vi "data-plotter.vi"() -> ()   [LabVIEW 2020]
uses:
  <vilib>/Utility/file.llb/Read Delimited Spreadsheet (DBL).vi
  <vilib>/Utility/file.llb/Read Delimited Spreadsheet (string).vi
panel:
  in  "文字列":string
  out "header row":string[](array[string]) caption="Header (1st row)"
  out "Graph":cluster{dbl[], dbl[]}(graph)
  in  "Y axis":i32
  in  "X axis":i32
  out "error out":errorcluster caption="エラー出力"
  in  "delimiter (\\t)":string="\t" caption="デリミタ (\\t)"
  in  "format (%.3f)":string="%.3f" caption="形式文字列 (%.3f)"
  in  "How many header rows?":i32
  in  "file path (dialog if empty)":path caption="ファイルパス (空の場合はダイアログ)"
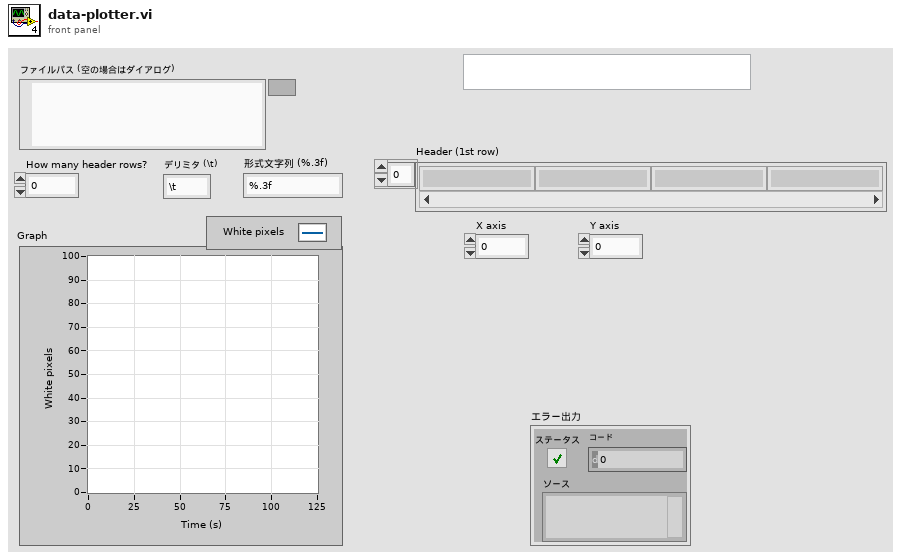
[diagram p1: front panel]
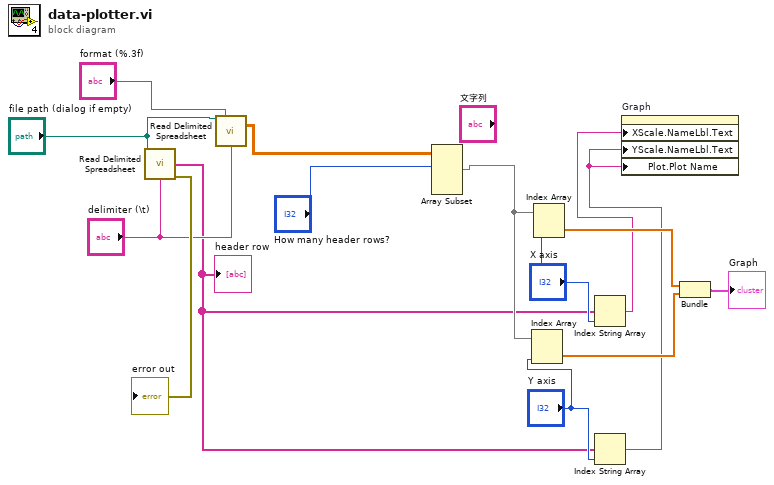
[diagram p0: block diagram]
diagram:
  n1 = call-poly <vilib>:"Read Delimited Spreadsheet.vi"("file path (dialog if empty)"="file path (dialog if empty)", "delimiter (\\t)"="delimiter (\\t)") -> ("first row"=w3:string[], "error out"=→"error out":errorcluster)  [unwired: 8 in, 4 out]
  "header row" <- w3
  n2 = call-poly <vilib>:"Read Delimited Spreadsheet.vi"("file path (dialog if empty)"="file path (dialog if empty)", "format (%.3f)"="format (%.3f)", "delimiter (\\t)"="delimiter (\\t)") -> ("all rows"=w6:dbl[][])  [unwired: 7 in, 5 out]
  n3 = Array Subset(array=w6, index (row)="How many header rows?") -> (w10:dbl[][])  [unwired: 3 in]
  n4 = Index Array(array=w10, index (col)="Y axis") -> (element=w12:dbl[])  [unwired: 1 in]
  n5 = Index Array(array=w10, index (col)="X axis") -> (element=w13:dbl[])  [unwired: 1 in]
  n6 = Index String Array(1:"X axis", 2:w3) -> (0:w2:string)  [unwired: 1 in]
  n7 = Index String Array(1:"Y axis", 2:w3) -> (0:w1:string)  [unwired: 1 in]
  n8 = property on="Graph" class="XYGraph (指定)"("XScale.NameLbl.Text"=w2, "YScale.NameLbl.Text"=w1, "Plot.Plot Name"=w1) -> ()  [unwired: 2 in, 2 out]
  n9 = Bundle(w13, w12) -> (→"Graph":cluster{dbl[], dbl[]})  [unwired: 1 in]
